vi "Initialize.vi"(8 "error in (no error)":errorcluster, 11 "Infiniium in":refnum<class "Infiniium.lvclass">) -> (0 "error out":errorcluster, 3 "Infiniium out":refnum<class "Infiniium.lvclass">)   [LabVIEW 2018, in "ScopePlugins.lvlib" / "Infiniium.lvclass"]
uses:
  Infiniium.lvclass
  C:/Users/ico/Documents/Projects/NistPluggableModules/Scope/ScopePlugins/ScopePluginBaseClass/ScopePluginsBase.lvclass
  ScopePluginBaseClass/ScopePluginsBase.lvclass/ScopePluginsBase.ctl
  ScopePluginBaseClass/Accessors/Write Channels.vi
  ScopePluginBaseClass/Accessors/Read Channels.vi
  <instrlib>/Agilent 90000 Series/Agilent 90000 Series.lvlib
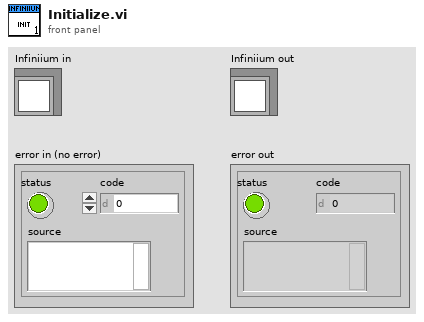
[diagram p1: front panel]
types:
  T1 = cluster{bool, "VISA resource name out":refnum<visa-resource-name>}[]
  T2 = typedef "ScopePlugins.lvlib/Channels.ctl" = cluster{"Count":i32, "ChannelArray":T3[]}
  T3 = typedef "ScopePlugins.lvlib/Channel.ctl" = cluster{"Enabled":bool, "Name":string, "InputImpedance":dbl, "InputFreqMax":dbl, "ProbeAttn":dbl, "Coupling":enum16{"AC", "DC", "GND"}, "Offset":dbl, "Range":dbl, "Handle":string, "Connected":bool, "Options String ":string}
  T4 = typedef "ScopePlugins.lvlib/InitOptions.ctl" = cluster{"Reset":bool, "IdQuery":bool, "AutoConfig":bool, "Options String":string, "Synchronize":bool}
  T5 = cluster{bool, "VISA resource name out":refnum<visa-resource-name>}
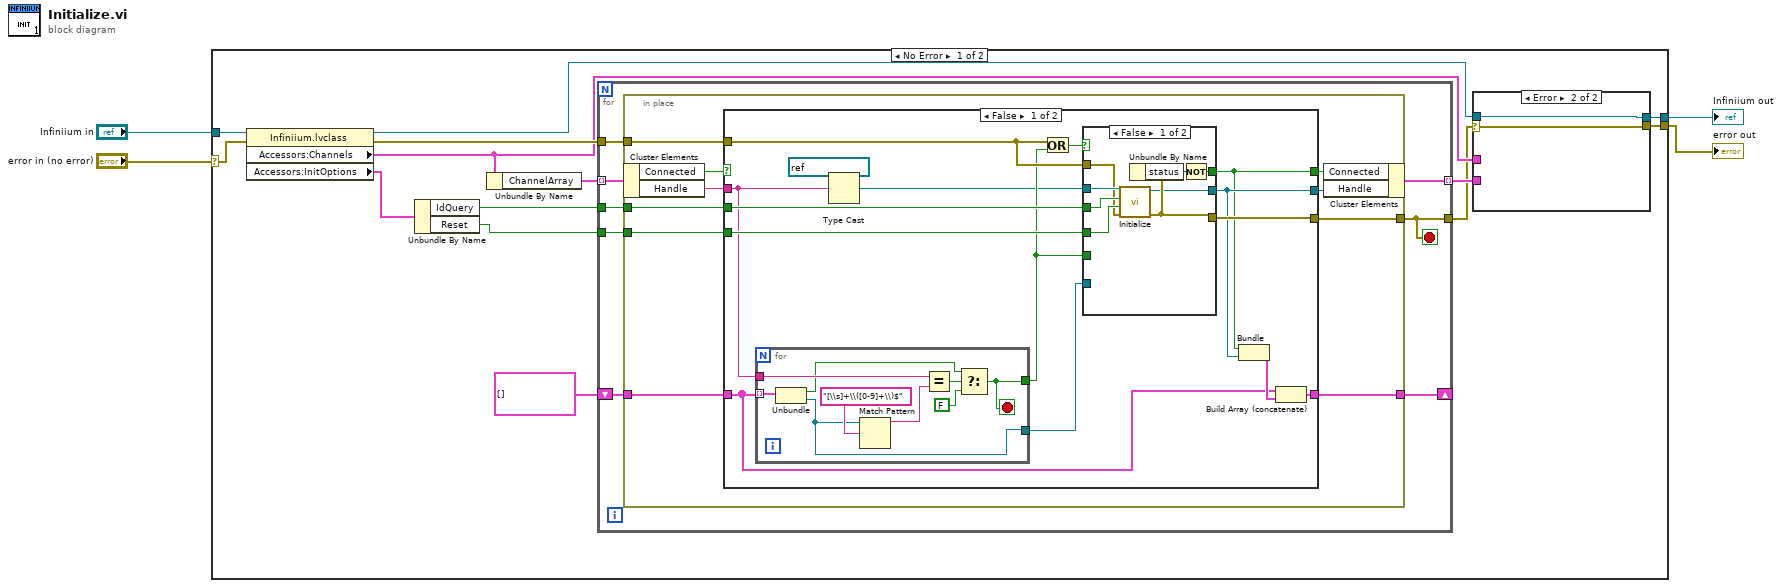
[diagram p0: block diagram]
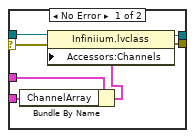
[diagram p2: hidden frame]
diagram:
  n1 = case shown="No Error" "error in (no error)" {
    selector: "error in (no error)" -> [w17 w85]
    tunnel: [w10 w86] -> w2
    tunnel: "Infiniium in" -> [w18 w86]
    tunnel: [w8 w85] -> w1
    frame No Error {
      n2 = property class="Infiniium.lvclass"(reference=w18, error in=w17) -> (reference out=w13:refnum<class "Infiniium.lvclass">, error out=w14:errorcluster, "Accessors:Channels"=w12:T2, "Accessors:InitOptions"=w7:T4)
      n3 = Unbundle By Name(w7) -> ("IdQuery"=w5:bool, "Reset"=w6:bool)
      n4 = Unbundle By Name(w12) -> ("ChannelArray"=w16:T3[])
      n5 = for {
        tunnel: w16 -> [w35] mode=indexing
        shift-right: [w29] -> _
        shift-left: T1 [] -> [w34]
        tunnel: w14 -> [w33]
        tunnel: w5 -> [w32]
        tunnel: w6 -> [w31]
        tunnel: [w30] -> w9
        tunnel: [w28] -> w11 mode=indexing
        stop <- w30 stop-if-true
        n6 = in-place {
          in-place-border: w34 -> [w45]
          in-place-border: w33 -> [w42]
          in-place-border: w32 -> [w41]
          in-place-border: w31 -> [w40]
          in-place-border: [w37] -> w30
          in-place-border: [w36] -> w29
          n7 = in-place-cluster #1(w35) -> ("Connected"=w44:bool, "Handle"=w43:string)
          n8 = case shown="False" w44 {
            selector: w44 -> [_ w84]
            tunnel: w45 -> [w50 w81]
            tunnel: w43 -> [w48 w83]
            tunnel: w42 -> [w57 w82]
            tunnel: w41 -> [w59 _]
            tunnel: w40 -> [w58 _]
            tunnel: [w56 w82] -> w37
            tunnel: [w53 w83] -> w39
            tunnel: [w52 w84] -> w38
            tunnel: [w49 w81] -> w36
            frame False {
              n9 = for {
                tunnel: w48 -> [w78]
                tunnel: [w75] -> w54
                tunnel: w50 -> [w74] mode=indexing
                tunnel: [w72] -> w55
                stop <- w75 stop-if-true
                n10 = Unbundle(w74) -> (w73:bool, "VISA resource name out"=w72:refnum<visa-resource-name>)
                n11 = Match Pattern(string=w72, regular expression="[\\s]+\\([0-9]+\\)$") -> (before substring=w79:string)  [unwired: 1 in, 3 out]
                n12 = Equal?(x=w78, y=w79) -> (x = y?=w77:bool)
                n13 = Select(t=w73, s=w77, f=FALSE) -> (s? t:f=w75:bool)
              }
              n14 = Type Cast(type=refnum<visa-resource-name> "DSOS104a" ("VISA resource name out"), x=w48) -> (*(type *) &x=w46:refnum<visa-resource-name>)
              n15 = Or(x=w57, y=w54) -> (x .or. y?=w60:bool)
              n16 = case shown="False" w60 {
                tunnel: w46 -> [w68 _]
                tunnel: w59 -> [w67 _]
                tunnel: w58 -> [w66 _]
                tunnel: w57 -> [w65 w71]
                tunnel: [w63 w71] -> w56
                tunnel: w55 -> [_ w70]
                tunnel: [w62 w70] -> w53
                tunnel: [w61 w69] -> w52
                tunnel: w54 -> [_ w69]
                frame False {
                  n17 = call <instrlib>:"Initialize.vi"("error in (no error)"=w65, "Reset (True)"=w66, "ID Query (True)"=w67, "VISA resource name"=w68) -> ("error out"=w63:errorcluster, "VISA resource name out"=w62:refnum<visa-resource-name>)  [unwired: 6 in]
                  n18 = Unbundle By Name(w63) -> ("status"=w64:bool)
                  n19 = Not(x=w64) -> (.not. x?=w61:bool)
                }
                frame True {
                }
              }
              n20 = Bundle(w52, "VISA resource name out"=w53) -> (w51:T5)  [unwired: 1 in]
              n21 = Build Array (concatenate)(w50, w51) -> (w49:T1)
            }
            frame True {
            }
          }
          n22 = in-place-cluster #1("Connected"=w38, "Handle"=w39) -> (w28:T3)
        }
      }
      n23 = case shown="Error" w9 {
        selector: w9 -> [w20 w26]
        tunnel: w13 -> [w25 w27]
        tunnel: w12 -> [w24 _]
        tunnel: w11 -> [w23 _]
        tunnel: [w21 w27] -> w10
        tunnel: [w19 w26] -> w8
        frame No Error {
          n24 = Bundle By Name(cluster=w24, "ChannelArray"=w23) -> (w22:T2)
          n25 = property class="Infiniium.lvclass"(reference=w25, error in=w20, "Accessors:Channels"=w22) -> (reference out=w21:refnum<class "Infiniium.lvclass">, error out=w19:errorcluster)
        }
        frame Error {
        }
      }
    }
    frame Error {
    }
  }
  "error out" <- w1
  "Infiniium out" <- w2
